vi "Handle Last Ack Core.vi"(4 "error in (no error)":errorcluster, 6 "Last Ack":refnum<class "Last Ack.lvclass">, 7 "User Interface in":refnum<class "User Interface.lvclass">) -> (0 "error out":errorcluster, 3 "User Interface out":refnum<class "User Interface.lvclass">)   [LabVIEW 2020, in "User Interface.lvlib" / "User Interface.lvclass"]
doc: "(<B>Filename</B>: Actor Framework.lvlib:Actor.lvclass:Handle Last Ack Core.vi)\n\nDefines how the caller actor responds to the Last Ack message from a nested actor. The Last Ack message is the final message a nested actor sends to its caller before it shuts down. The message contains information about the final state of the nested actor.\n\nBy default, this method does nothing except return any error the nested actor sent. A descendant class may override this method to define behavior."
uses:
  User Interface.lvclass
  <vilib>/ActorFramework/LastAck/Last Ack.lvclass
  <vilib>/ActorFramework/LastAck/Last Ack.lvclass/Last Ack.ctl
  <vilib>/ActorFramework/Actor/Actor.lvclass
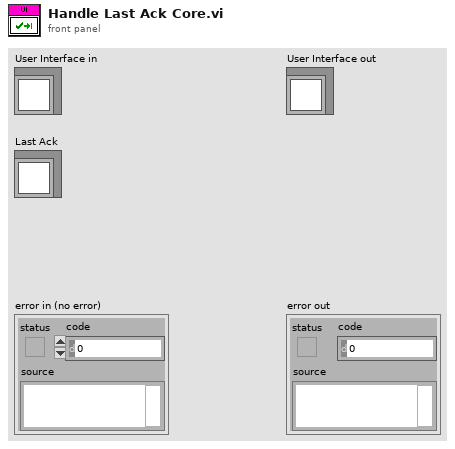
[diagram p1: front panel]
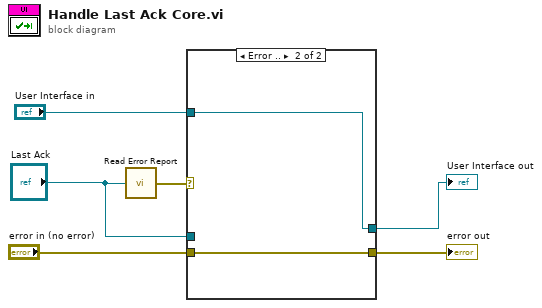
[diagram p0: block diagram]
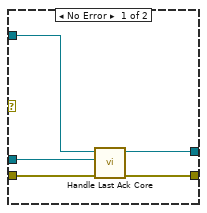
[diagram p2: hidden frame]
diagram:
  n1 = call <vilib>:"Read Error Report.vi"("Last Ack"="Last Ack") -> ("error report"=w1:errorcluster)
  n2 = case shown="Error .." w1 {
    tunnel: [w11 w12] -> w6
    tunnel: [w10 w13] -> w5
    tunnel: "error in (no error)" -> [w9 w12]
    tunnel: "User Interface in" -> [w8 w13]
    tunnel: "Last Ack" -> [w7 _]
    frame No Error {
      n3 = call-parent "Handle Last Ack Core.vi"("error in (no error)"=w9, "Last Ack"=w7, "Actor in"=w8) -> ("error out"=w11:errorcluster, "Actor out"=w10:refnum<class "User Interface.lvclass">)  [unwired: 3 in]
    }
    frame Error {
    }
  }
  "User Interface out" <- w5
  "error out" <- w6
